vi "FGV CAN 2.vi"(6 "Aktion":T8, 7 "CAN Data":T1=[{"timestamp"=timestamp(0 s since 1904-01-01), "payload"=[0, 2, 3, 4, 5, 6, 7, 8], "identifier"=2, "type"=0, "extended?"=FALSE, "echo?"=FALSE}, {"timestamp"=timestamp(0 s since 1904-01-01), "payload"=[0, 1, 2, 3, 4, 5, 6, 7], "identifier"=3, "type"=0, "extended?"=FALSE, "echo?"=FALSE}] {"payload" format="%x"; "timestamp" format="%<%.7X\n%x>T"; "type" items=["CAN Data"=0, "CAN Remote"=1, "CAN Bus Error"=2, "CAN 2.0 Data"=8, "CAN FD Data"=16, "CAN FD+BRS Data"=24, "J1939 Data"=192, "Delay"=224, "Log Trigger"=225, "Start Trigger"=226]; "identifier" format="%x"}, 8 "error in (no error)":errorcluster caption="Fehler (Eingang, kein Fehler)", 10 "selected SAE J-1939 Signals In":refnum<k21>[](array[refnum]), 11 "Konfig Daten":T7={"Baude Rate"=500000, "COM state"=0, "Interface"="CAN1"} {"Baude Rate" items=["40 kBaud"=40000, "50 kBaud"=50000, "62,5 kBaud"=62500, "80 kBaud"=80000, "83,3 kBaud"=83300, "100 kBaud"=100000, "125 kBaud"=125000, "160 kBaud"=160000, "200 kBaud"=200000, "250 kBaud"=250000, "400 kBaud"=400000, "500 kBaud"=500000, "800 kBaud"=800000, "1 MBaud"=1000000]}) -> (0 "error out":errorcluster caption="Fehler (Ausgang)", 1 "Messwerte":dbl[](array[numeric]), 2 "selected SAE J-1939 Signals Out":refnum<k21>[](array[refnum]), 3 "Konfig Daten":T7={"Baude Rate"=250000, "COM state"=0, "Interface"="CAN1"} {"Baude Rate" items=["40 kBaud"=40000, "50 kBaud"=50000, "62,5 kBaud"=62500, "80 kBaud"=80000, "83,3 kBaud"=83300, "100 kBaud"=100000, "125 kBaud"=125000, "160 kBaud"=160000, "200 kBaud"=200000, "250 kBaud"=250000, "400 kBaud"=400000, "500 kBaud"=500000, "800 kBaud"=800000, "1 MBaud"=1000000]}, 4 "DBC DB-Cluster":T5, 5 "CAN Data out":T4={"CAN Data selected"=[{"timestamp"=timestamp(0 s since 1904-01-01), "payload"=[0, 2, 3, 4, 5, 6, 7, 8], "identifier"=2, "type"=0, "extended?"=FALSE, "echo?"=FALSE}, {"timestamp"=timestamp(0 s since 1904-01-01), "payload"=[0, 1, 2, 3, 4, 5, 6, 7], "identifier"=3, "type"=0, "extended?"=FALSE, "echo?"=FALSE}], "more CAN Data"=[{"timestamp"=timestamp(0 s since 1904-01-01), "payload"=[0, 2, 3, 4, 5, 6, 7, 8], "identifier"=2, "type"=0, "extended?"=FALSE, "echo?"=FALSE}, {"timestamp"=timestamp(0 s since 1904-01-01), "payload"=[0, 1, 2, 3, 4, 5, 6, 7], "identifier"=3, "type"=0, "extended?"=FALSE, "echo?"=FALSE}]} {"more CAN Data"."payload" format="%x"; "more CAN Data"."timestamp" format="%<%.7X\n%x>T"; "more CAN Data"."type" items=["CAN Data"=0, "CAN Remote"=1, "CAN Bus Error"=2, "CAN 2.0 Data"=8, "CAN FD Data"=16, "CAN FD+BRS Data"=24, "J1939 Data"=192, "Delay"=224, "Log Trigger"=225, "Start Trigger"=226]; "more CAN Data"."identifier" format="%x"; "CAN Data selected"."payload" format="%x"; "CAN Data selected"."timestamp" format="%<%.7X\n%x>T"; "CAN Data selected"."type" items=["CAN Data"=0, "CAN Remote"=1, "CAN Bus Error"=2, "CAN 2.0 Data"=8, "CAN FD Data"=16, "CAN FD+BRS Data"=24, "J1939 Data"=192, "Delay"=224, "Log Trigger"=225, "Start Trigger"=226]; "CAN Data selected"."identifier" format="%x"})   [LabVIEW 2020, in "CAN Konfig.lvlib"]
uses:
  CAN Konfig.lvlib
  Aktion FGV CAN2.ctl
  cRIO/CAN Interface/Baude Rate.ctl
  cRIO/CAN Interface/CAN Data.ctl
  <vilib>/xnet/xnet.llb/XNET Frame CAN.ctl
  <vilib>/xnet/xnet.llb/XNET Frame Type CAN.ctl
  <vilib>/xnet/xnet.llb/XNET Database Close (Signal).vi
  Allgemein/allgemeine Sub-VIs.lvlib
  cRIO/CAN Interface/CAN Interface.lvlib
panel:
  in  "Status":u32[](array[numeric])
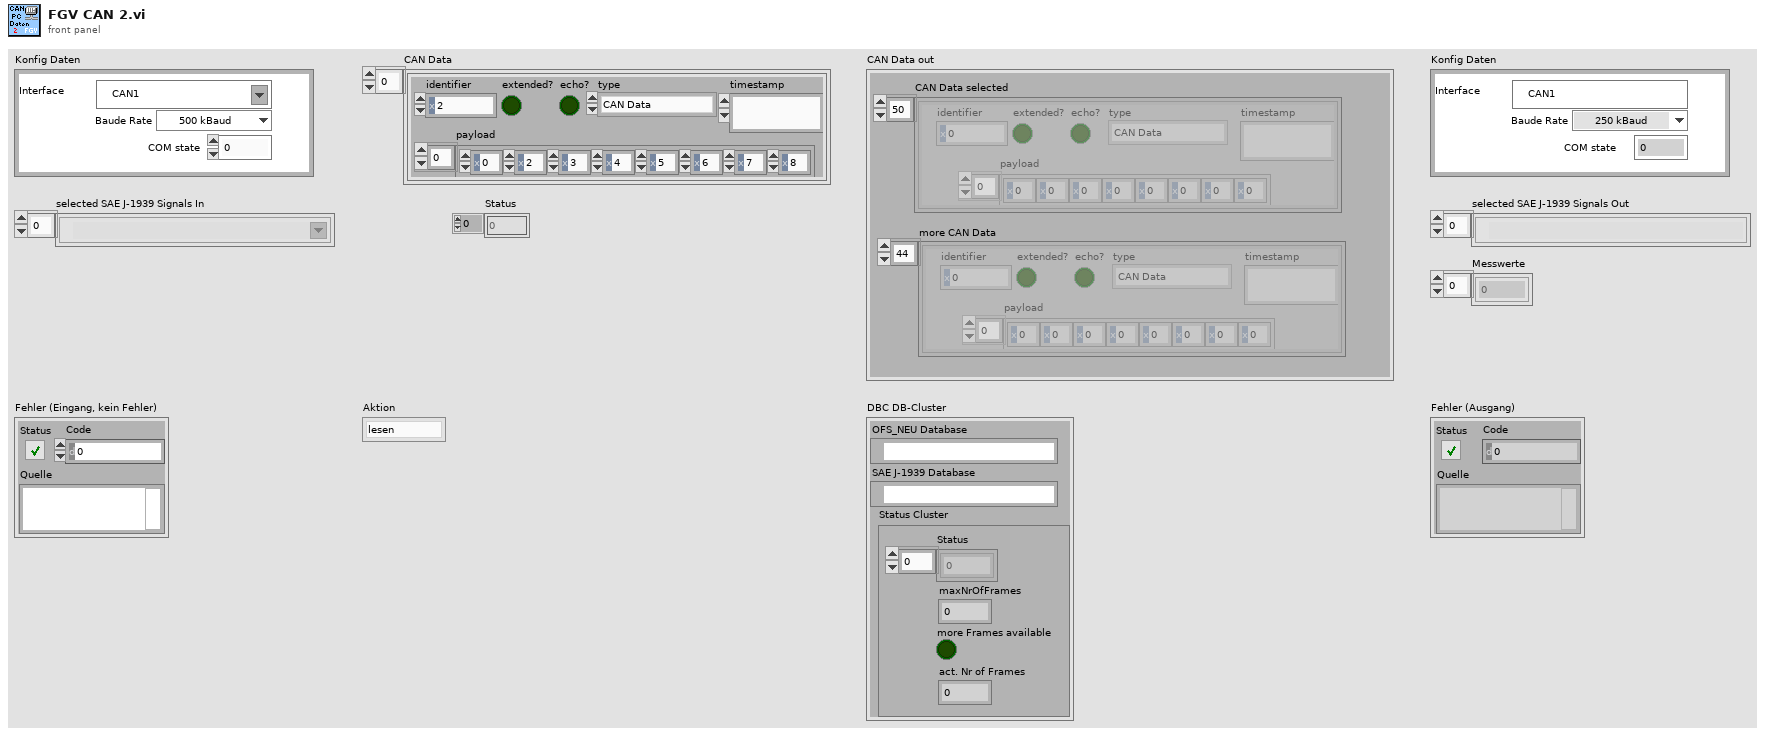
[diagram p1: front panel]
types:
  T1 = typedef "CAN Interface.lvlib/CAN Data.ctl" = T2[]
  T2 = typedef "XNET Frame CAN.ctl" = cluster{"timestamp":timestamp, "payload":u8[], "identifier":u32, "type":T3, "extended?":bool, "echo?":bool}
  T3 = typedef "XNET Frame Type CAN.ctl" = u8
  T4 = cluster{"CAN Data selected":T1, "more CAN Data":T1}
  T5 = cluster{"OFS_NEU Database":refnum<k21>, "SAE J-1939 Database":refnum<k21>, "Status Cluster":cluster{"Status":u32[], "maxNrOfFrames":i32, "more Frames available":bool, "act. Nr of Frames":i32}}
  T6 = typedef "CAN Interface.lvlib/Baude Rate.ctl" = u32
  T7 = cluster{"Baude Rate":T6, "COM state":u8, "Interface":refnum<k21>}
  T8 = typedef "CAN Konfig.lvlib/Aktion FGV CAN2.ctl" = enum16{"lesen", "schreiben Konfig", "Status", "Messdaten", "laden", "speichern", "CAN Data", "reset more Frames avalable"}
  T9 = cluster{"SAE J-1939 Database":refnum<k21>, "XNET Database":refnum<k21>, cluster{"Status":u32[], i32, bool, i32}}
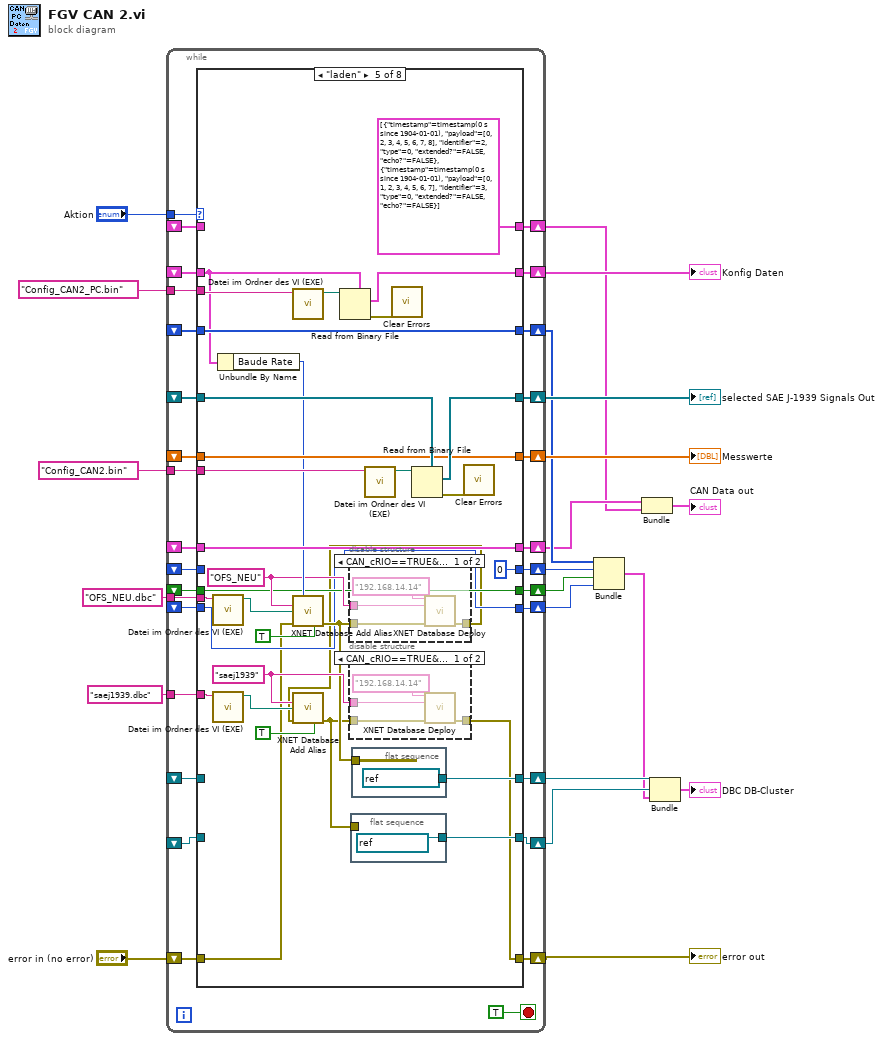
[diagram p0: block diagram]
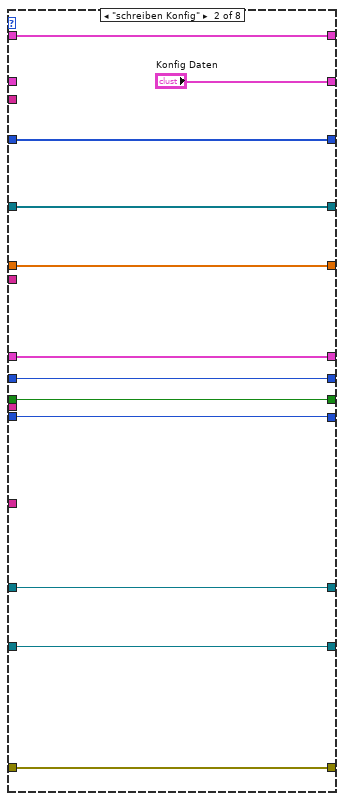
[diagram p3: hidden frame]
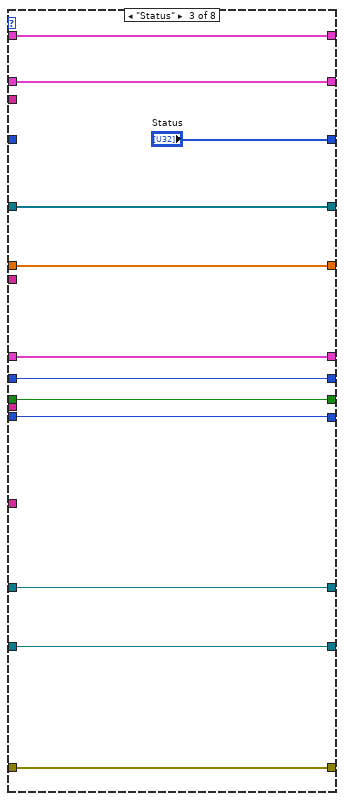
[diagram p4: hidden frame]
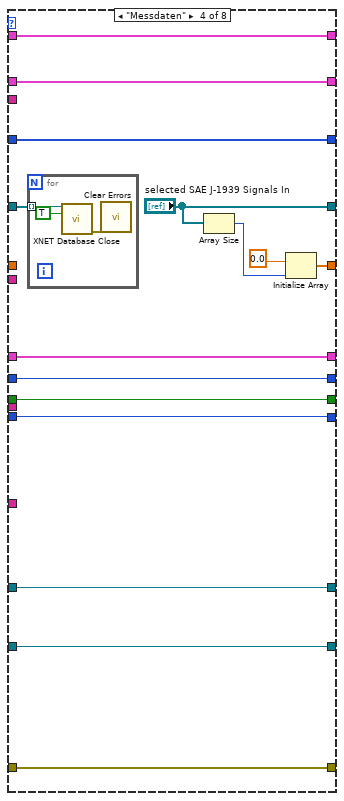
[diagram p5: hidden frame]
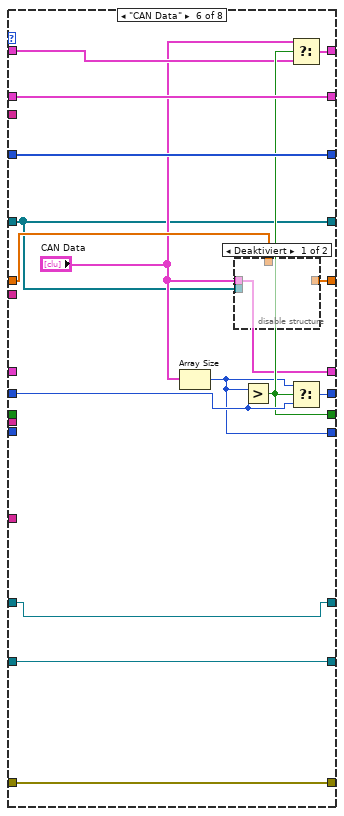
[diagram p8: hidden frame]
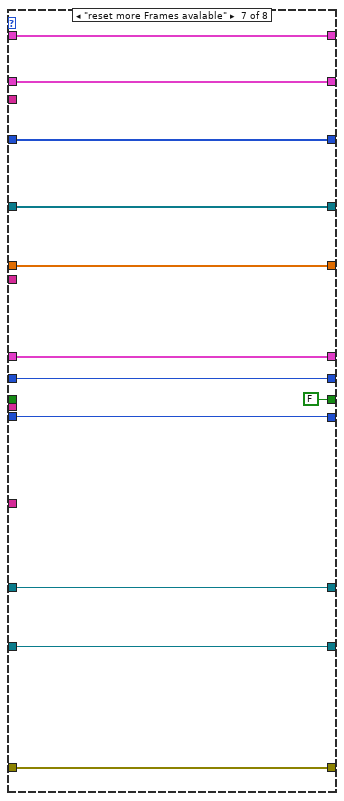
[diagram p10: hidden frame]
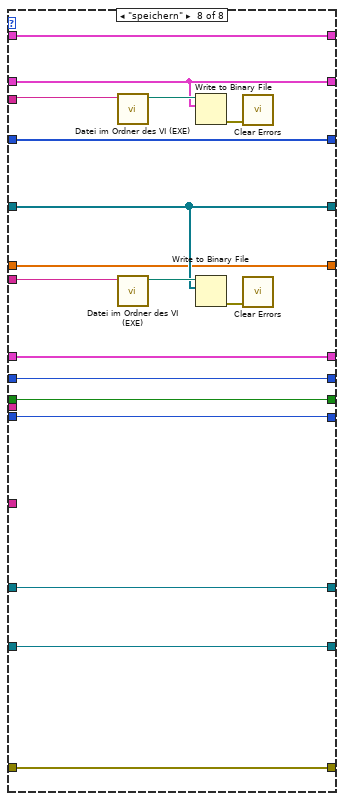
[diagram p11: hidden frame]
diagram:
  n1 = while {
    tunnel: "Aktion" -> [w50]
    shift-right: [w49] -> w20
    shift-left: _ -> [w47]
    shift-right: [w48] -> w8
    shift-left: _ -> [w46]
    shift-right: [w45] -> w19
    shift-left: _ -> [w44]
    tunnel: "Config_CAN2.bin" ("Dateiname") -> [w43]
    shift-right: [w42] -> w6
    shift-left: _ -> [w41]
    tunnel: "Config_CAN2_PC.bin" ("Dateiname") -> [w40]
    shift-right: [w39] -> w15
    shift-left: _ -> [w38]
    shift-right: [w37] -> w11
    shift-left: _ -> [w36]
    shift-right: [w35] -> w16
    shift-left: _ -> [w34]
    tunnel: "OFS_NEU.dbc" ("Dateiname") -> [w33]
    tunnel: "saej1939.dbc" ("Dateiname") -> [w32]
    shift-right: [w31] -> w9
    shift-left: _ -> [w30]
    shift-right: [w29] -> w10
    shift-left: _ -> [w28]
    shift-right: [w27] -> w5
    shift-left: _ -> [w26]
    shift-right: [w25] -> w3
    shift-left: _ -> [w24]
    shift-right: [w22] -> w1
    shift-left: "error in (no error)" -> [w23]
    stop <- TRUE stop-if-true
    n2 = case shown="\"laden\"" w50 {
      tunnel: [w60 "Konfig Daten" w84 w100 w129 w164 w181 w191] -> w49
      tunnel: [w63 w75 "Status" w102 w138 w165 w180 w199] -> w48
      tunnel: w47 -> [w60 _ w84 w100 w121 w164 w181 w191]
      tunnel: w46 -> [w63 w75 _ w102 w138 w165 w180 w199]
      tunnel: [w62 w74 w86 "selected SAE J-1939 Signals In" w135 w151 w179 w197] -> w45
      tunnel: w44 -> [w62 w74 w86 w97 w134 w151 w179 w197]
      tunnel: w43 -> [_ _ _ _ w137 _ _ w195]
      tunnel: [w61 w73 w85 w101 w132 "CAN Data" w173 w194] -> w42
      tunnel: w41 -> [w61 w73 w85 w101 w132 _ w173 w194]
      tunnel: w40 -> [_ _ _ _ w130 _ _ w190]
      tunnel: [w59 w71 w83 w99 w127 w163 w178 w189] -> w39
      tunnel: w38 -> [w59 w71 w83 w99 _ w163 w178 w189]
      tunnel: [w58 w70 w82 w94 w126 w160 w177 w188] -> w37
      tunnel: w36 -> [w58 w70 w82 _ w126 w161 w177 w188]
      tunnel: [w57 w69 w81 w98 w125 w162 w176 w187] -> w35
      tunnel: w34 -> [w57 w69 w81 w98 _ w162 w176 w187]
      tunnel: w33 -> [_ _ _ _ w124 _ _ _]
      tunnel: w32 -> [_ _ _ _ w115 _ _ _]
      tunnel: [w56 w68 w80 w92 0 w158 w175 w186] -> w31
      tunnel: w30 -> [w56 w68 w80 w92 _ w159 w175 w186]
      tunnel: [w55 w67 w79 w91 w112 w157 FALSE w185] -> w29
      tunnel: w28 -> [w55 w67 w79 w91 w112 _ _ w185]
      tunnel: [w54 w66 w78 w90 T1 [{"timestamp"=timestamp(0 s since 1904-01-01), "payload"=[0, 2, 3, 4, 5, 6, 7, 8], "identifier"=2, "type"=0, "extended?"=FALSE, "echo?"=FALSE}, {"timestamp"=timestamp(0 s since 1904-01-01), "payload"=[0, 1, 2, 3, 4, 5, 6, 7], "identifier"=3, "type"=0, "extended?"=FALSE, "echo?"=FALSE}] ("CAN Data") w156 w172 w184] -> w27
      tunnel: w26 -> [w54 w66 w78 w90 _ w155 w172 w184]
      tunnel: [w53 w65 w77 w89 w110 w154 w171 w183] -> w25
      tunnel: w24 -> [w53 w65 w77 w89 w110 _ w171 w183]
      tunnel: w23 -> [w52 w64 w76 w88 w108 w153 w170 w182]
      tunnel: [w52 w64 w76 w88 w106 w153 w170 w182] -> w22
      frame "lesen", Default {
      }
      frame "schreiben Konfig" {
      }
      frame "Status" {
      }
      frame "Messdaten" {
        n3 = for {
          tunnel: w97 -> [w105] mode=indexing
          n4 = call-poly <vilib>:"XNET Database Close.vi"("signal in"=w105, "close all? (true)"=TRUE) -> ("error out"=w103:errorcluster)  [unwired: 13 in]
          n5 = call <vilib>:"Clear Errors.vi"("error in (no error)"=w103) -> ()  [unwired: 5 in, 2 out]
        }
        n6 = Array Size(array="selected SAE J-1939 Signals In") -> (size(s)=w95:i32)
        n7 = Initialize Array(0.0 ("value"), w95) -> (w94:dbl[])
      }
      frame "laden" {
        w118 = "saej1939" ("alias")
        w119 = "OFS_NEU" ("alias")
        n8 = call "Datei im Ordner des VI (EXE).vi"("Dateiname"=w124) -> ("Dateipfad im Ordner des Haupt-VIs"=w123:path)  [unwired: 8 in, 2 out]
        n9 = call "Datei im Ordner des VI (EXE).vi"("Dateiname"=w115) -> ("Dateipfad im Ordner des Haupt-VIs"=w116:path)  [unwired: 8 in, 2 out]
        n10 = Unbundle By Name(w121) -> ("Baude Rate"=w120:T6)
        n11 = call "Datei im Ordner des VI (EXE).vi"("Dateiname"=w130) -> ("Dateipfad im Ordner des Haupt-VIs"=w128:path)  [unwired: 8 in, 2 out]
        n12 = call <vilib>:"XNET Database Add Alias.vi"("default baud rate (0)"=w120, "alias"=w119, "filepath"=w123, "error in (no error)"=w108, "ignore application protocol (F)"=TRUE) -> ("error out"=w114:errorcluster)  [unwired: 10 in]
        n13 = Read from Binary File(5:w121, 11:w128) -> (0:w131:errorcluster, 2:w129:T7)  [unwired: 1 in, 5 out]
        n14 = disable-structure shown="CAN_cRIO==TRUE&&cRio_aktiv==TRUE" {
          disable-tunnel: w114 -> [w149 w150]
          disable-tunnel: [w148 w150] -> w107
          disable-tunnel: w119 -> [w147 _]
          frame condition #0 {
            n15 = call <vilib>:"XNET Database Deploy.vi"("IP address"="192.168.14.14" ("IP Adresse"), "alias"=w147, "error in (no error)"=w149) -> ("error out"=w148:errorcluster)  [unwired: 11 in, 1 out]
          }
          frame condition #1 (active) {
          }
        }
        n16 = call <vilib>:"XNET Database Add Alias.vi"("alias"=w118, "filepath"=w116, "error in (no error)"=w107, "ignore application protocol (F)"=TRUE) -> ("error out"=w113:errorcluster)  [unwired: 11 in]
        n17 = disable-structure shown="CAN_cRIO==TRUE&&cRio_aktiv==TRUE" {
          disable-tunnel: w113 -> [w144 w145]
          disable-tunnel: [w143 w145] -> w106
          disable-tunnel: w118 -> [w142 _]
          frame condition #0 {
            n18 = call <vilib>:"XNET Database Deploy.vi"("IP address"="192.168.14.14" ("IP Adresse"), "alias"=w142, "error in (no error)"=w144) -> ("error out"=w143:errorcluster)  [unwired: 11 in, 1 out]
          }
          frame condition #1 (active) {
          }
        }
        n19 = flat-sequence {
          tunnel: [refnum<k21> "saej1939" ("XNET Database")] -> w127
          tunnel: w113 -> [_]
          frame #0 {
          }
        }
        n20 = flat-sequence {
          tunnel: [refnum<k21> "OFS_NEU" ("SAE J-1939 Database")] -> w125
          tunnel: w114 -> [_]
          frame #0 {
          }
        }
        n21 = call "Datei im Ordner des VI (EXE).vi"("Dateiname"=w137) -> ("Dateipfad im Ordner des Haupt-VIs"=w136:path)  [unwired: 8 in, 2 out]
        n22 = call <vilib>:"Clear Errors.vi"("error in (no error)"=w131) -> ()  [unwired: 5 in, 2 out]
        n23 = Read from Binary File(5:w134, 11:w136) -> (0:w133:errorcluster, 2:w135:refnum<k21>[])  [unwired: 1 in, 5 out]
        n24 = call <vilib>:"Clear Errors.vi"("error in (no error)"=w133) -> ()  [unwired: 5 in, 2 out]
      }
      frame "CAN Data" {
        n25 = Array Size(array="CAN Data") -> (size(s)=w154:i32)
        n26 = disable-structure shown="Deaktiviert" {
          disable-tunnel: w161 -> [w168 w169]
          disable-tunnel: [_ w169] -> w160
          disable-tunnel: "CAN Data" -> [w167 _]
          disable-tunnel: w151 -> [w166 _]
          frame Disabled {
          }
          frame Enabled {
          }
        }
        n27 = Greater?(x=w154, y=w159) -> (0:w157:bool)
        n28 = Select(t="CAN Data", s=w157, f=w155) -> (s? t:f=w156:T1)
        n29 = Select(t=w154, s=w157, f=w159) -> (s? t:f=w158:i32)
      }
      frame "reset more Frames avalable" {
      }
      frame "speichern" {
        n30 = call "Datei im Ordner des VI (EXE).vi"("Dateiname"=w190) -> ("Dateipfad im Ordner des Haupt-VIs"=w192:path)  [unwired: 8 in, 2 out]
        n31 = call "Datei im Ordner des VI (EXE).vi"("Dateiname"=w195) -> ("Dateipfad im Ordner des Haupt-VIs"=w198:path)  [unwired: 8 in, 2 out]
        n32 = Write to Binary File(file (use dialog)=w192, data=w191) -> (error out=w193:errorcluster)  [unwired: 1 in, 5 out]
        n33 = Write to Binary File(file (use dialog)=w198, data=w197) -> (error out=w196:errorcluster)  [unwired: 1 in, 5 out]
        n34 = call <vilib>:"Clear Errors.vi"("error in (no error)"=w193) -> ()  [unwired: 5 in, 2 out]
        n35 = call <vilib>:"Clear Errors.vi"("error in (no error)"=w196) -> ()  [unwired: 5 in, 2 out]
      }
    }
  }
  "Konfig Daten" <- w20
  "error out" <- w1
  "selected SAE J-1939 Signals Out" <- w19
  "Messwerte" <- w11
  n36 = Bundle("Status"=w8, w9, w10, w3) -> (w7:cluster{"Status":u32[], i32, bool, i32})  [unwired: 1 in]
  n37 = Bundle("CAN Data"=w6, "CAN Data"=w5) -> (→"CAN Data out":cluster{"CAN Data":T1, "CAN Data":T1})  [unwired: 1 in]
  n38 = Bundle("SAE J-1939 Database"=w16, "XNET Database"=w15, w7) -> (→"DBC DB-Cluster":T9)  [unwired: 1 in]
